vi "RP instrument test.vi"() -> ()   [LabVIEW 2016]
uses:
  RP Instrument.lvclass
  RP Instrument.lvclass/RP Instrument.ctl
  Write Status check delay.vi
  Write DDS delay.vi
  Write Decimation.vi
  Write Post-trigger samples.vi
panel:
  in  "Frequency":dbl=100.0 format="%#_6p"
  in  "Post-trigger points":i32=10000
  in  "Pre-trigger points":i32=1000
  in  "Decimation":i32=64
  in  "Status check delay":u32=6
  in  "DDS delay":u32=47
  out "Waveform Graph 2":i16[](graph)
  in  "Number WFRM points":i32=1000000 format="%.0p"
  out "Waveform Graph":i16[][](graph)
  in  "Reset":bool=TRUE
  in  "read size":i32=300
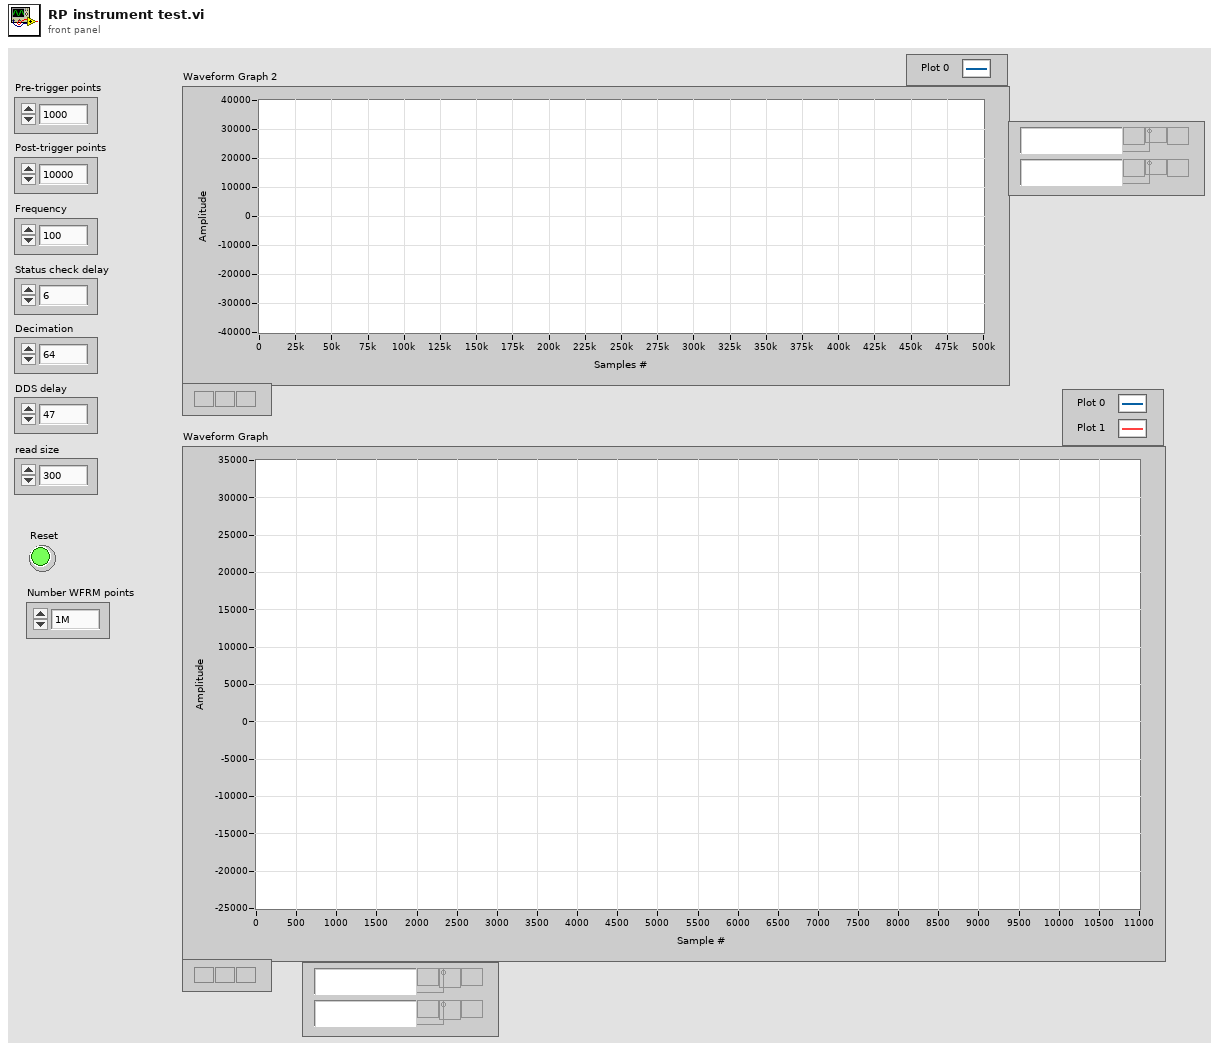
[diagram p1: front panel]
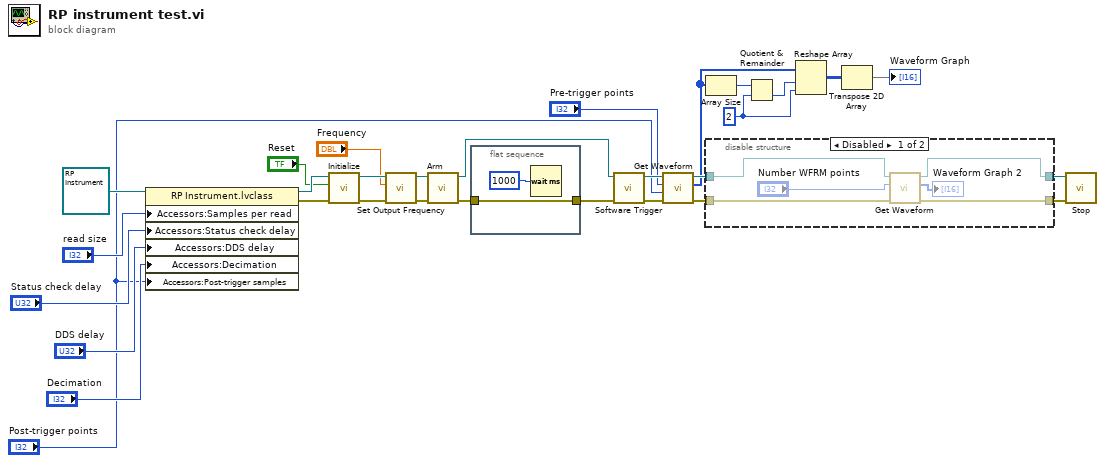
[diagram p0: block diagram]
diagram:
  w3 = 2 ("dimension size")
  n1 = property class="RP Instrument.lvclass"(reference=refnum<class "RP Instrument.lvclass"> refnum ("RP Instrument.lvclass"), "Accessors:Samples per read"="read size", "Accessors:Status check delay"="Status check delay", "Accessors:DDS delay"="DDS delay", "Accessors:Decimation"="Decimation", "Accessors:Post-trigger samples"="Post-trigger points") -> (reference out=w30:refnum<class "RP Instrument.lvclass">, error out=w29:errorcluster)  [unwired: 1 in]
  n2 = call-dynamic "Initialize.vi"("error in (no error)"=w29, "Reset"="Reset", "RP Instrument in"=w30) -> ("error out"=w5:errorcluster, "RP Instrument out"=w26:refnum<class "RP Instrument.lvclass">)  [unwired: 7 in]
  n3 = call-dynamic "Set Output Frequency.vi"("error in (no error)"=w5, "Frequency"="Frequency", "RP Instrument in"=w26) -> ("error out"=w4:errorcluster, "RP Instrument out"=w7:refnum<class "RP Instrument.lvclass">)  [unwired: 7 in]
  n4 = call-dynamic "Arm.vi"("error in (no error)"=w4, "RP Instrument in"=w7) -> ("error out"=w10:errorcluster, "RP Instrument out"=w11:refnum<class "RP Instrument.lvclass">)  [unwired: 8 in]
  n5 = flat-sequence {
    tunnel: w10 -> [w32]
    tunnel: [w32] -> w13
    frame #0 {
      n6 = Wait (ms)(milliseconds to wait=u32 1000) -> ()  [unwired: 1 out]
    }
  }
  n7 = call-dynamic "Software Trigger.vi"("error in (no error)"=w13, "RP Instrument in"=w11) -> ("error out"=w12:errorcluster, "RP Instrument out"=w14:refnum<class "RP Instrument.lvclass">)  [unwired: 8 in]
  n8 = call-dynamic "Get Waveform.vi"("error in (no error)"=w12, "Post-trigger points"="Post-trigger points", "Pre-trigger points"="Pre-trigger points", "RP Instrument in"=w14) -> ("error out"=w23:errorcluster, "Data out"=w16:i16[], "RP Instrument out"=w28:refnum<class "RP Instrument.lvclass">)  [unwired: 5 in]
  n9 = Array Size(array=w16) -> (size(s)=w15:i32)
  n10 = disable-structure shown="Disabled" {
    disable-tunnel: w28 -> [w38 w39]
    disable-tunnel: [w37 w39] -> w24
    disable-tunnel: w23 -> [w34 w40]
    disable-tunnel: [w33 w40] -> w22
    frame Disabled {
      n11 = call-dynamic "Get Waveform.vi"("error in (no error)"=w34, "Pre-trigger points"="Number WFRM points", "RP Instrument in"=w38) -> ("error out"=w33:errorcluster, "Data out"=→"Waveform Graph 2":i16[], "RP Instrument out"=w37:refnum<class "RP Instrument.lvclass">)  [unwired: 6 in]
    }
    frame Enabled {
    }
  }
  n12 = Quotient & Remainder(x=w15, y=w3) -> (floor(x/y)=w2:i32)  [unwired: 1 out]
  n13 = Reshape Array(w16, w2, w3) -> (w17:i16[][])
  n14 = Transpose 2D Array(2D array=w17) -> (transposed array=→"Waveform Graph":i16[][])
  n15 = call-dynamic "Stop.vi"("error in (no error)"=w22, "RP Instrument in"=w24) -> ()  [unwired: 8 in, 2 out]
